vi "sub_Enqueue.vi"(10 "commands":T1[](array[typedef]), 11 "queue":refnum<queue>) -> ()   [LabVIEW 2018]
uses:
  TicTacToeControl.ctl
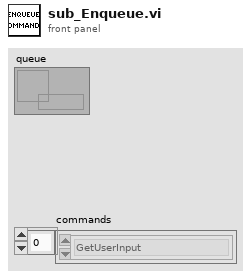
[diagram p1: front panel]
types:
  T1 = typedef "TicTacToeControl.ctl" = enum16{"Initialize", "GetUserInput", "GetComputerMove", "SetControlValue", "Initialize Control References", "Wait for player move", "Quit", "Play Again ?", "Check result "}
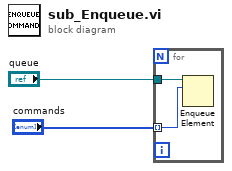
[diagram p0: block diagram]
diagram:
  n1 = for {
    tunnel: "queue" -> [w4]
    tunnel: "commands" -> [w3] mode=indexing
    n2 = Enqueue Element(queue=w4, element=w3) -> ()  [unwired: 2 in, 3 out]
  }
